vi "4461 - AI AND AI - Read AND Write Uneven - SINGLE TASK.vi"(6 "Write":waveform(dbl)[](array[waveform]), 8 "error in (no error)":errorcluster, 9 "sampling info":cluster{"Fs":dbl, "#s":dbl}={"Fs"=1000.0, "#s"=1000.0} {"Fs" format="%.2p"}, 10 "AO task":refnum<k21>, 11 "AI task":refnum<k21>) -> (0 "error out":errorcluster, 3 "Read":waveform(dbl)[](array[waveform]))   [LabVIEW 2016]
uses:
  <vilib>/DAQmx/write.llb/DAQmx Write (Analog 1D Wfm NChan NSamp).vi
  <vilib>/DAQmx/read.llb/DAQmx Read (Analog 1D Wfm NChan NSamp).vi
  <vilib>/DAQmx/miscellaneous.llb/DAQmx Fill In Error Info.vi
  <resource>/objmgr/daqmx.rc
panel:
  out "Numeric":i32
  out "AvailSampPerChan":u32
  # "OUTPUTS"
  # "INPUTS"
  # "These are just for debugging / monitoring"
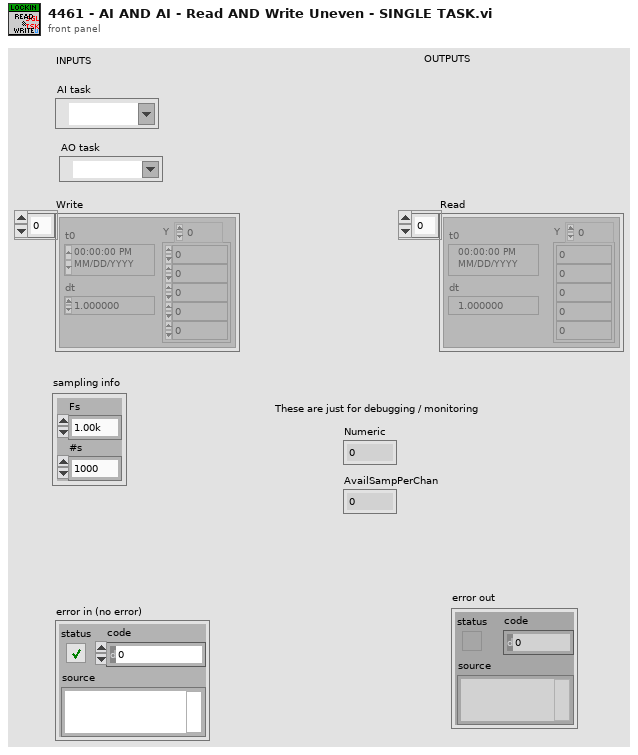
[diagram p1: front panel]
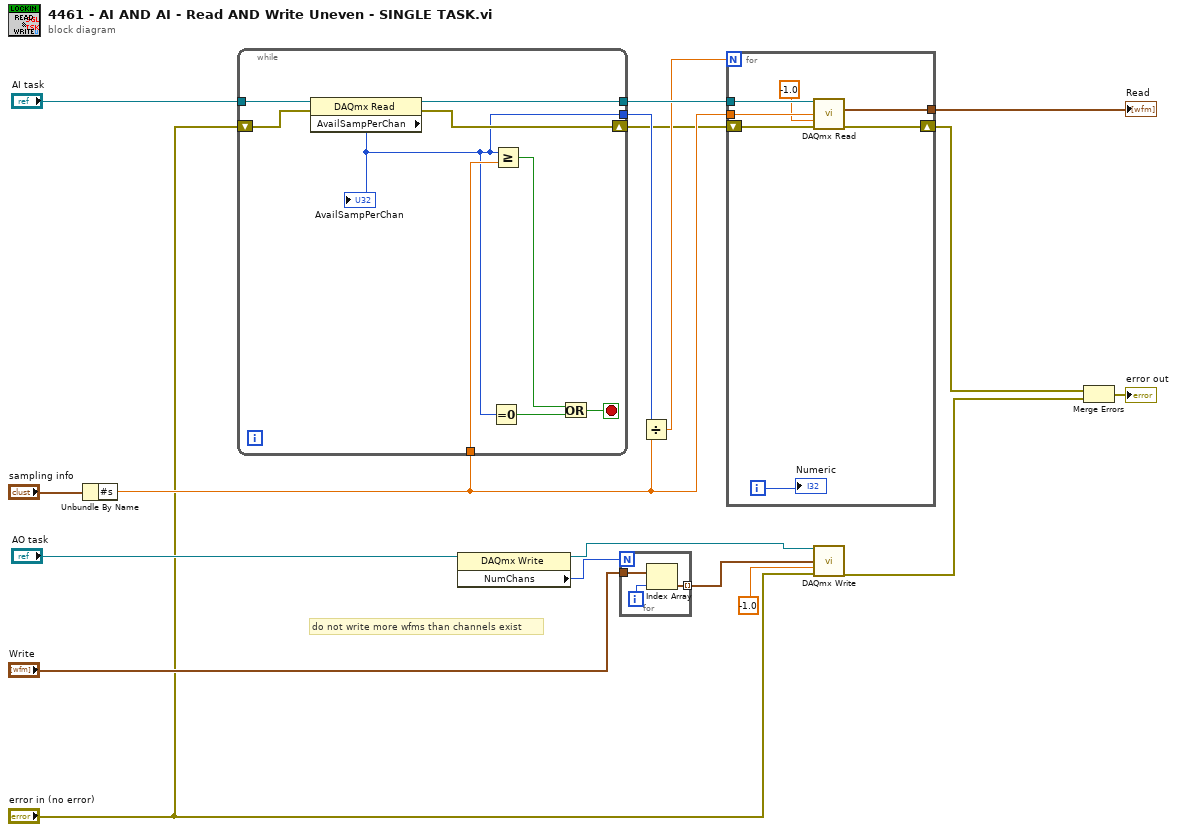
[diagram p0: block diagram]
diagram:
  # "do not write more wfms than channels exist"
  n1 = Unbundle By Name("sampling info") -> ("#s"=w16:dbl)
  n2 = while {
    tunnel: [w27] -> w15
    tunnel: w16 -> [w25]
    tunnel: [w20] -> w13
    tunnel: "AI task" -> [w21]
    shift-right: [w26] -> w4
    shift-left: "error in (no error)" -> [w19]
    stop <- w24 stop-if-true
    n3 = property class="DAQmx Read"(reference=w21, error in=w19) -> (reference out=w27:refnum<k21>, error out=w26:errorcluster, "AvailSampPerChan"=w20:u32)
    "AvailSampPerChan" <- w20
    n4 = Equal To 0?(x=w20) -> (x = 0?=w23:bool)
    n5 = Greater Or Equal?(x=w20, y=w25) -> (x >= y?=w22:bool)
    n6 = Or(x=w22, y=w23) -> (x .or. y?=w24:bool)
  }
  n7 = property class="DAQmx Write"(reference="AO task") -> (reference out=w8:refnum<k21>, "NumChans"=w12:u32)  [unwired: 1 in, 1 out]
  n8 = for {
    N: w12 -> [_]
    tunnel: "Write" -> [w30]
    tunnel: [w29] -> w11 mode=indexing
    i -> [w28]
    n9 = Index Array(array=w30, index=w28) -> (element=w29:waveform(dbl))
  }
  n10 = Divide(x=w13, y=w16) -> (x/y=w14:dbl)
  n11 = for {
    N: w14 -> [_]
    tunnel: w15 -> [w37]
    tunnel: [w36] -> w5
    tunnel: w16 -> [w35]
    shift-right: [w34] -> w2
    shift-left: w4 -> [w31]
    i -> [w33]
    n12 = call-poly <vilib>:"DAQmx Read.vi"("task/channels in"=w37, "number of samples per channel"=w35, "timeout"=-1.0, "error in"=w31) -> ("data"=w36:waveform(dbl)[], "error out"=w34:errorcluster)  [unwired: 9 in, 1 out]
    "Numeric" <- w33
  }
  "Read" <- w5
  n13 = call-poly <vilib>:"DAQmx Write.vi"("task/channels in"=w8, "data"=w11, "timeout"=-1.0, "error in"="error in (no error)") -> ("error out"=w1:errorcluster)  [unwired: 9 in, 2 out]
  n14 = Merge Errors(w2, w1) -> (→"error out":errorcluster)
